vi "FT10_Config Parse File.vi"(8 "error in (no error)":errorcluster, 10 "File Path Control":path=path "Config.ini") -> (0 "error out":errorcluster, 2 "Config cluster":T2={"Unitherm Port"="COM4", "Simulate Values"=TRUE, "Fornax Connect Attempts"=0})   [LabVIEW 2015]
doc: "Open \"Config.ini\" file and bundle key values into config cluster"
uses:
  Controls/Control_Config Unitherm Found Bool.ctl
  Controls/Control_Config Simulation Found Bool.ctl
  Controls/Control_Config Cluster.ctl
  Controls/Control_Config Unitherm Port.ctl
  Controls/Control_Config Simulate Values.ctl
  Controls/Control_Config Fornax Connect Attempts.ctl
  Controls/Control_Config Fornax Attempts Found Bool.ctl
  <vilib>/Utility/config.llb/Read Key (String).vi
  <vilib>/Utility/config.llb/NI_LVConfig.lvlib
panel:
  out "Fornax Attempts found?":T1
  out "Simulation found?":T6=TRUE
  out "Unitherm found?":T7=TRUE
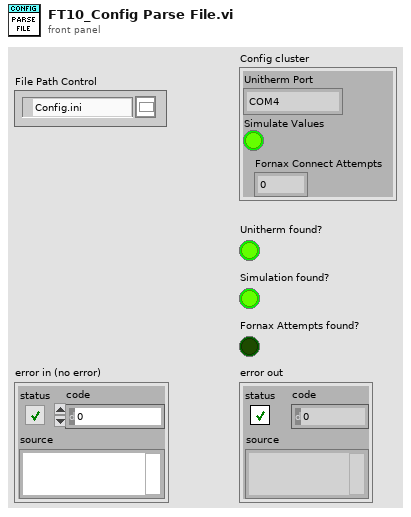
[diagram p1: front panel]
types:
  T1 = typedef "Control_Config Fornax Attempts Found Bool.ctl" = bool
  T2 = typedef "Control_Config Cluster.ctl" = cluster{"Unitherm Port":T3, "Simulate Values":T4, "Fornax Connect Attempts":T5}
  T3 = typedef "Control_Config Unitherm Port.ctl" = string
  T4 = typedef "Control_Config Simulate Values.ctl" = bool
  T5 = typedef "Control_Config Fornax Connect Attempts.ctl" = i32
  T6 = typedef "Control_Config Simulation Found Bool.ctl" = bool
  T7 = typedef "Control_Config Unitherm Found Bool.ctl" = bool
  T8 = typedef "NI_LVConfig.lvlib/Config Data RefNum.ctl" = refnum<k1>
  T9 = typedef "Control_Config Str Val Cluster.ctl" = cluster{"Unitherm value":T10, "Simulation value":T11, "Fornax Attempts value":T12}
  T10 = typedef "Control_Config Unitherm Str Val.ctl" = string
  T11 = typedef "Control_Config Simulation Str Val.ctl" = string
  T12 = typedef "Control_Config Fornax Attempts Str Val.ctl" = string
  T13 = typedef "Control_Config Keys Found Cluster.ctl" = cluster{"Unitherm found?":T7, "Simulation found?":T6, "Fornax Attempts found?":T1}
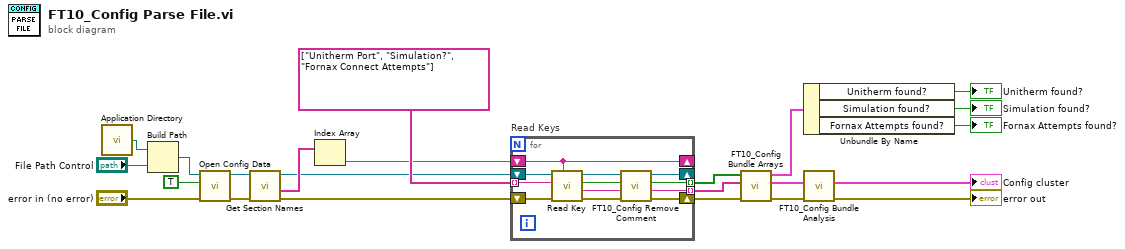
[diagram p0: block diagram]
diagram:
  n1 = call <vilib>:"Application Directory.vi"() -> ("Application Directory"=w17:path)
  n2 = Build Path(base path=w17, name or relative path="File Path Control") -> (appended path=w23:path)
  n3 = call <vilib>:"Open Config Data.vi"("error in (no error)"="error in (no error)", "create file if necessary (T)"=TRUE, "configuration file path"=w23) -> ("error out"=w16:errorcluster, "refnum"=w18:T8)  [unwired: 6 in, 1 out]
  n4 = call <vilib>:"Get Section Names.vi"("error in (no error)"=w16, "refnum"=w18) -> ("error out"=w20:errorcluster, "section names"=w22:string[], "refnum out"=w19:T8)  [unwired: 7 in]
  n5 = Index Array(array=w22) -> (element=w12:string)  [unwired: 1 in]
  n6 = for "Read Keys" {
    tunnel: [w25] -> w6 mode=indexing
    tunnel: [w26] -> w11 mode=indexing
    tunnel: string[] ["Unitherm Port", "Simulation?", "Fornax Connect Attempts"] ("key") -> [w35] mode=indexing
    shift-right: [w24] -> w5
    shift-left: w20 -> [w34]
    shift-right: [w32] -> _
    shift-left: w12 -> [w32]
    shift-right: [w27] -> _
    shift-left: w19 -> [w33]
    n7 = call-poly <vilib>:"Read Key.vi"("section"=w32, "error in (no error)"=w34, "key"=w35, "refnum"=w33) -> ("error out"=w28:errorcluster, "value"=w29:string, "found?"=w30:bool, "refnum out"=w31:T8)  [unwired: 4 in]
    n8 = call "FT10_Config Remove Comment.vi"("error in"=w28, "Value In"=w29, "found? in"=w30, "refnum in"=w31) -> ("error out"=w24:errorcluster, "Value without Comment"=w25:string, "found? out"=w26:bool, "refnum out"=w27:T8)  [unwired: 4 in]
  }
  n9 = call "FT10_Config Bundle Arrays.vi"("error in (no error)"=w5, "String Values Array"=w6, "Values Found Array"=w11) -> ("error out"=w2:errorcluster, "Config String Value Cluster"=w4:T9, "Config Keys Found Cluster"=w10:T13)  [unwired: 6 in]
  n10 = Unbundle By Name(w10) -> ("Unitherm found?"=→"Unitherm found?":T7, "Simulation found?"=→"Simulation found?":T6, "Fornax Attempts found?"=→"Fornax Attempts found?":T1)
  n11 = call "FT10_Config Bundle Analysis.vi"("error in (no error)"=w2, "Config String Value Cluster"=w4) -> ("error out"=→"error out":errorcluster, "Config cluster"=→"Config cluster":T2)  [unwired: 8 in]
